vi "LibXML_NodeToAttributePointer.vi"(8 "error in":errorcluster, 11 "node  in":u32) -> (0 "error out":errorcluster, 3 "attr out":u32)   [LabVIEW 2019, in "Tools.lvlib" / "LibXML.lvlib"]
doc: "Gets a pointer (U32) to the attributes of a node"
uses:
  LibXML.lvlib
  dll/lXMLwrap.dll
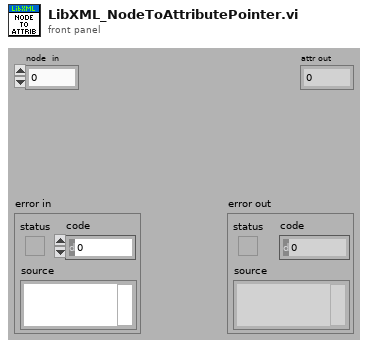
[diagram p1: front panel]
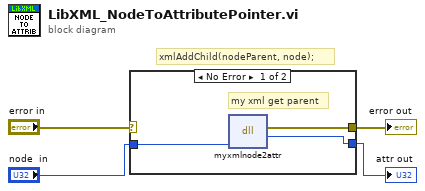
[diagram p0: block diagram]
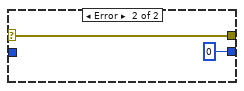
[diagram p2: hidden frame]
diagram:
  # "xmlAddChild(nodeParent, node);"
  n1 = case shown="No Error" "error in" {
    selector: "error in" -> [_ w9]
    tunnel: [w5 w9] -> w3
    tunnel: [w7 u32 0 ("return type")] -> w2
    tunnel: "node  in" -> [w6 _]
    frame No Error {
      # "my xml get parent"
      n2 = dll-call lib="C:/Projects/_Prywatne/MyCIT/Framework/Tools/XML/LibXML/dll/lXMLwrap.dll" fn="myxmlnode2attr"("node"=w6) -> (error out=w5:errorcluster, "return type"=w7:u32)  [unwired: 4 in, 1 out]
    }
    frame Error {
    }
  }
  "error out" <- w3
  "attr out" <- w2
